vi "LSX Set Controller.vi"(6 "lAC":i32, 7 "lZC":i32, 8 "error in (no error)":errorcluster, 9 "lYC":i32, 10 "lXC":i32, 11 "lLSID":i32) -> (0 "error out":errorcluster, 3 "function return":i32)   [LabVIEW 2016, in "Tango_DLL.lvlib"]
doc: "TANGOAPI int TANGOCALL LSX_SetController (int lLSID, int lXC, int lYC, int lZC, int lAC);"
uses:
  Tango_DLL.lvlib
  2017/Microscope Control/Device Library/Stages/Marzhauser/SCAN IM 120 x 80/Tango DLL VIs/Tango_DLL.dll
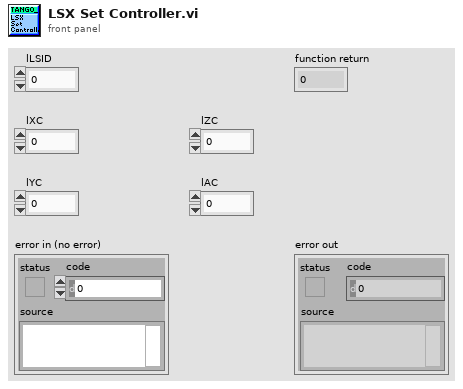
[diagram p1: front panel]
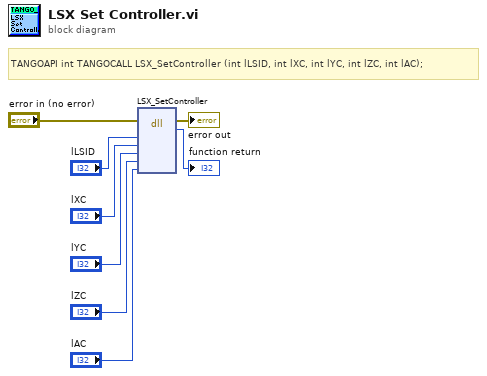
[diagram p0: block diagram]
diagram:
  # "TANGOAPI int TANGOCALL LSX_SetController (int lLSID, int lXC, int lYC, int lZC, int lAC);"
  n1 = dll-call lib="C:/Users/4PiSMS/Documents/Microscope Control/2017/Microscope Control/Device Library/Stages/Marzhauser/SCAN IM 120 x 80/Tango DLL VIs/Tango_DLL.*" fn="LSX_SetController"(error in="error in (no error)", "lLSID"="lLSID", "lXC"="lXC", "lYC"="lYC", "lZC"="lZC", "lAC"="lAC") -> (error out=→"error out":errorcluster, →"function return":i32)  [unwired: 7 in, 1 out]
